vi "Test_RouteGuide_BidirectionalStreaming.vi"() -> (0 "Array of Error Description":T1)   [LabVIEW 2019]
uses:
  gRPC_ATS/TestUtility/utility.llb/array of error description.ctl
  gRPC_ATS/TestUtility/utility.llb/error description.ctl
  gRPC_ATS/TestUtility/utility.llb/error type.ctl
  examples/route_guide/route_guide_client/RPC Messages/routeguide_RouteNote.ctl
  examples/route_guide/route_guide_client/RPC Messages/routeguide_Point.ctl
  examples/route_guide/route_guide_client/route_guide_client.lvlib
panel:
  out "Pass":bool
  in  "Client VI Path":path=path "../../examples/route_guide/route_guide_client/Bidirectional Streaming RouteGuide Test.vi"
  in  "Server VI path":path=path "../../examples/route_guide/route_guide_server/Run Service.vi"
  in  "error in":errorcluster
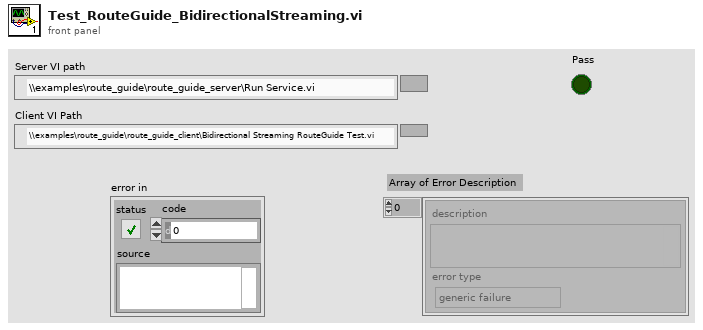
[diagram p1: front panel]
types:
  T1 = typedef "array of error description.ctl" = T2[]
  T2 = typedef "error description.ctl" = cluster{"description":string, "error type":T3}
  T3 = typedef "error type.ctl" = enum32{"generic failure", "boundary case", "precision", "expected error"}
  T4 = typedef "route_guide_client.lvlib/routeguide_RouteNote.ctl" = cluster{"location":T5, "message":string}
  T5 = typedef "route_guide_client.lvlib/routeguide_Point.ctl" = cluster{"latitude":i32, "longitude":i32}
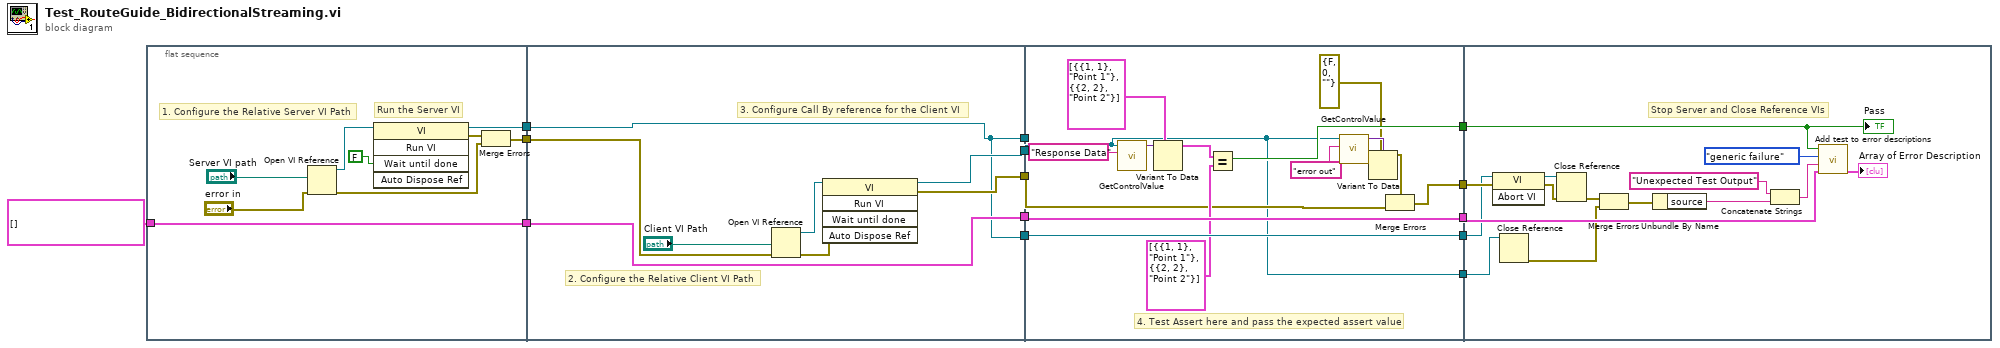
[diagram p0: block diagram]
diagram:
  n1 = flat-sequence {
    tunnel: T1 [] ("error descriptions in") -> [w19]
    tunnel: [w19] -> w14
    tunnel: [w18] -> w13
    tunnel: [w15] -> w12
    tunnel: w14 -> [w30]
    tunnel: [w30] -> w11
    tunnel: [w24] -> w10
    tunnel: w13 -> [w24]
    tunnel: w12 -> [w29]
    tunnel: [w24] -> w5
    tunnel: [w26] -> w3
    tunnel: [w25] -> w2
    tunnel: w11 -> [w46]
    tunnel: [w46] -> w9
    tunnel: [w34] -> w8
    tunnel: w10 -> [_]
    tunnel: [w44] -> w6
    tunnel: w5 -> [w45]
    tunnel: [w45] -> w4
    tunnel: w3 -> [w38]
    tunnel: w2 -> [w32]
    tunnel: [w32] -> w1
    tunnel: w9 -> [w56]
    tunnel: w8 -> [w53]
    tunnel: w6 -> [w52]
    tunnel: w4 -> [w48]
    tunnel: w1 -> [w47]
    frame #0 {
      # "1. Configure the Relative Server VI Path"
      # "Run the Server VI"
      n2 = Open VI Reference(vi path="Server VI path", error in (no error)="error in") -> (vi reference=w21:refnum<vi>, error out=w17:errorcluster)  [unwired: 4 in]
      n3 = invoke class="VI" method="Run VI"(reference=w21, "Wait until done"=FALSE ("Wait Until Done")) -> (reference out=w18:refnum<vi>, error out=w16:errorcluster)  [unwired: 3 in, 3 out]
      n4 = Merge Errors(w16, w17) -> (w15:errorcluster)
    }
    frame #1 {
      # "2. Configure the Relative Client VI Path"
      # "3. Configure Call By reference for the Client VI"
      n5 = Open VI Reference(vi path="Client VI Path", error in (no error)=w29) -> (vi reference=w27:refnum<vi>, error out=w28:errorcluster)  [unwired: 4 in]
      n6 = invoke class="VI" method="Run VI"(reference=w27, error in=w28) -> (reference out=w25:refnum<vi>, error out=w26:errorcluster)  [unwired: 3 in, 3 out]
    }
    frame #2 {
      # "4. Test Assert here and pass the expected assert value"
      n7 = call "GetControlValue.vi"("Control Label"="Response Data", "VI Reference"=w32) -> ("Value"=w42:variant)  [unwired: 8 in, 1 out]
      n8 = Variant To Data(type=T4[] [{"location"={"latitude"=1, "longitude"=1}, "message"="Point 1"}, {"location"={"latitude"=2, "longitude"=2}, "message"="Point 2"}] ("Response Data"), Variant=w42) -> (data=w40:T4[])  [unwired: 1 in, 1 out]
      n9 = Equal?(x=w40, y=T4[] [{"location"={"latitude"=1, "longitude"=1}, "message"="Point 1"}, {"location"={"latitude"=2, "longitude"=2}, "message"="Point 2"}] ("Response Data")) -> (x = y?=w44:bool)
      n10 = call "GetControlValue.vi"("Control Label"="error out", "VI Reference"=w32) -> ("Value"=w36:variant)  [unwired: 8 in, 1 out]
      n11 = Variant To Data(type=errorcluster {"status"=FALSE, "code"=0, "source"=""} ("error constant"), Variant=w36) -> (data=w33:errorcluster)  [unwired: 1 in, 1 out]
      n12 = Merge Errors(w33, w38) -> (w34:errorcluster)
    }
    frame #3 {
      # "Stop Server and Close Reference VIs"
      n13 = invoke class="VI" method="Abort VI"(reference=w48, error in=w53) -> (reference out=w54:refnum<vi>, error out=w55:errorcluster)  [unwired: 1 in, 1 out]
      n14 = Close Reference(reference=w47) -> (error out=w50:errorcluster)  [unwired: 1 in]
      n15 = Close Reference(reference=w54, error in (no error)=w55) -> (error out=w51:errorcluster)
      n16 = Merge Errors(w51, w50) -> (w49:errorcluster)
      n17 = Unbundle By Name(w49) -> ("source"=w58:string)
      n18 = Concatenate Strings("Unexpected Test Output" ("string"), w58) -> (w59:string)
      n19 = call "Add test to error descriptions.vi"("error descriptions in"=w56, "error string"=w59, "error type"=error_type."generic failure", "pass"=w52) -> ("error description out"=→"Array of Error Description":T1)  [unwired: 3 in]
      "Pass" <- w52
    }
  }
